vi "Freeze Value.vi"(0 "Input":dbl, 2 "Freeze Value":bool) -> (20 "Output":dbl)   [LabVIEW 2019]
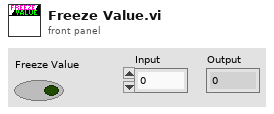
[diagram p1: front panel]
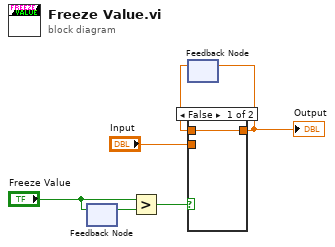
[diagram p0: block diagram]
diagram:
  n1 = feedback #1() -> (w6:bool)  [unwired: 1 in]
  n2 = feedback-in #1("Freeze Value") -> ()
  n3 = Greater?(x="Freeze Value", y=w6) -> (0:w4:bool)
  n4 = feedback #2() -> (w3:dbl)  [unwired: 1 in]
  n5 = case shown="False" w4 {
    tunnel: [w7 w8] -> w1
    tunnel: w3 -> [w7 _]
    tunnel: "Input" -> [_ w8]
    frame False {
    }
    frame True {
    }
  }
  "Output" <- w1
  n6 = feedback-in #2(w1) -> ()
